vi "libssh2_knownhost_get - invalid known hosts collection - eol reached is true.vi"() -> ()   [LabVIEW 2013, in "libssh2_tests.lvlib"]
uses:
  libssh2_tests.lvlib
  libssh2/Known Hosts Collection Refnum.ctl
  libssh2/libssh2_init (Default).vi
  <vilib>/addons/_JKI Toolkits/Caraya/classes/Assert/Assert True.vi
  <vilib>/addons/_JKI Toolkits/Caraya/classes/Test/Test.lvclass
  libssh2/libssh2.lvlib
  <vilib>/addons/_JKI Toolkits/Caraya/classes/Assert/Assert.lvclass
panel:
  out "error out":errorcluster
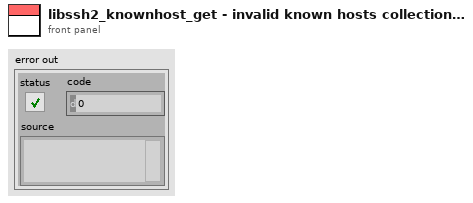
[diagram p1: front panel]
types:
  T1 = typedef "libssh2.lvlib/Known Hosts Collection Refnum.ctl" = refnum<k1>
  T2 = typedef "libssh2.lvlib/Session Refnum.ctl" = refnum<k1>
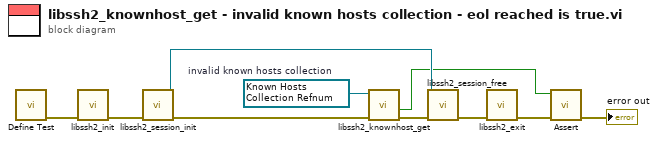
[diagram p0: block diagram]
diagram:
  w3 = T1 refnum items=["Known Hosts"]  # invalid known hosts collection
  n1 = call <vilib>:"Define Test.vi"() -> ("error out"=w9:errorcluster)  [unwired: 10 in, 1 out]
  n2 = call-poly "libssh2_init.vi"("error in (no error)"=w9) -> ("error out"=w8:errorcluster)  [unwired: 10 in]
  n3 = call "libssh2_session_init.vi"("error in (no error)"=w8) -> ("error out"=w4:errorcluster, "session"=w5:T2)  [unwired: 9 in]
  n4 = call "libssh2_knownhost_get.vi"("error in (no error)"=w4, "known hosts collection"=w3) -> ("error out"=w1:errorcluster, "end reached"=w2:bool)  [unwired: 7 in, 1 out]
  n5 = call "libssh2_session_free.vi"("error in (no error)"=w1, "session"=w5) -> ("error out"=w7:errorcluster)  [unwired: 9 in]
  n6 = call "libssh2_exit.vi"("error in (no error)"=w7) -> ("error out"=w6:errorcluster)  [unwired: 10 in]
  n7 = call-poly <vilib>:"Assert.vi"("error in (no error)"=w6, "True?"=w2) -> ("error out"=→"error out":errorcluster)  [unwired: 8 in, 1 out]
